vi "Get I2C Channels.vi"(8 "Error In":errorcluster, 11 "LINX Device Config":T1) -> (0 "Error Out":errorcluster, 1 "Num Channels":u8, 2 "I2C Channels":u8[](array[numeric]), 3 "LINX Device Config":T1)   [LabVIEW 2014, in "LMH-LINX.lvlib" / "Device.lvlib"]
uses:
  <vilib>/MakerHub/LINX/Private/Device/Device.lvlib
  <vilib>/MakerHub/LINX/Private/Device/Type Defs/LINX Device Config.ctl
  <vilib>/MakerHub/LINX/Private/Type Defs/Interface.ctl
  <vilib>/MakerHub/LINX/Private/Device/Type Defs/TCP Config.ctl
  <vilib>/MakerHub/LINX/Private/Device/Type Defs/Channels.ctl
  <vilib>/MakerHub/LINX/Private/Type Defs/Error Type.ctl
  <vilib>/MakerHub/LINX/LMH-LINX.lvlib
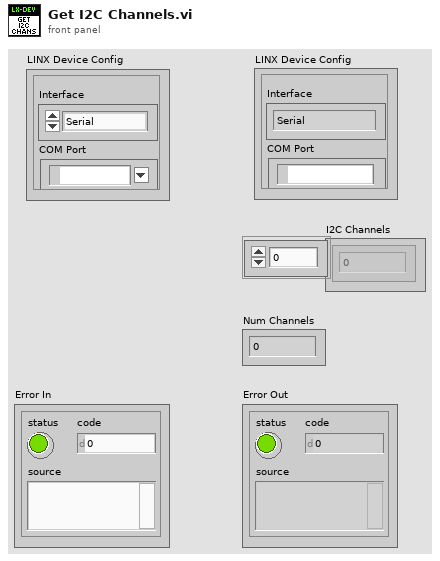
[diagram p1: front panel]
types:
  T1 = typedef "LMH-LINX.lvlib/Device.lvlib/LINX Device Config.ctl" = cluster{"Interface":T2, "COM Port":refnum<visa-resource-name>, "TCP Configuration":T3, "Device Family":u8, "Device ID":u8, "Device Name":string, "TCP Ref":refnum<k5>, "Channels":T4}
  T2 = typedef "LMH-LINX.lvlib/Interface.ctl" = enum16{"Serial", "TCP"}
  T3 = typedef "LMH-LINX.lvlib/Device.lvlib/TCP Config.ctl" = cluster{"IP Address":string, "Port":u16}
  T4 = typedef "LMH-LINX.lvlib/Channels.ctl" = cluster{"DI":u8[], "DO":u8[], "AI":u8[], "AO":u8[], "PWM":u8[], "QE":u8[], "UART":u8[], "I2C 2":u8[], "SPI":u8[], "CAN":u8[], "Servo":u8[], "AI Ref (V)":dbl, "AI Resolution (Bits)":u8, "AO Ref (V)":dbl, "AO Resolution (Bits)":u8}
  T5 = typedef "LMH-LINX.lvlib/Error Type.ctl" = enum16{"Unknown", "Timeout", "Corrupt Return Packet", "Unable To Connect", "Command Not Supported", "Channel DNE", "Invalid COM Config", "Firmware Version Mismatch", "myRIO Support", "CMD Specific Error", "Local IO Not Supported"}
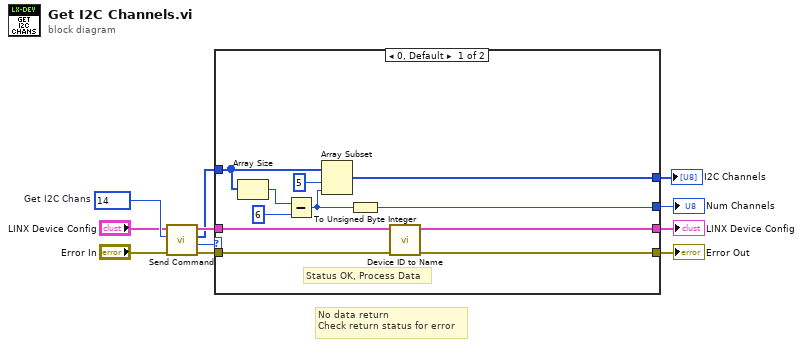
[diagram p0: block diagram]
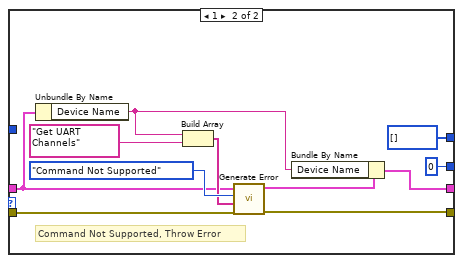
[diagram p2: hidden frame]
diagram:
  w10 = u16 14  # Get I2C Chans
  # "No data return\nCheck return status for error"
  n1 = call <vilib>:"Send Command.vi"("Error In"="Error In", "CMD"=w10, "LINX Device Config"="LINX Device Config") -> ("Error Out"=w5:errorcluster, "Status"=w3:u8, "Response"=w4:u8[], "LINX Device Config"=w7:T1)  [unwired: 5 in]
  n2 = case shown="0, Default" w3 {
    tunnel: [w19 w27] -> w8
    tunnel: w7 -> [w22 w26]
    tunnel: [w20 w32] -> w6
    tunnel: w5 -> [w21 w33]
    tunnel: w4 -> [w18 _]
    tunnel: [w14 u8[] []] -> w2
    tunnel: [w12 u8 0] -> w1
    frame 0, Default {
      # "Status OK, Process Data"
      n3 = Array Size(array=w18) -> (size(s)=w17:i32)
      n4 = Subtract(x=w17, y=6 ("index")) -> (x-y=w13:i32)
      n5 = Array Subset(array=w18, index=5, length=w13) -> (w14:u8[])
      n6 = To Unsigned Byte Integer(number=w13) -> (unsigned 8bit integer=w12:u8)
      n7 = call <vilib>:"Device ID to Name.vi"("Error In"=w21, "LINX Device Config"=w22) -> ("Error Out"=w20:errorcluster, "LINX Device Config"=w19:T1)  [unwired: 7 in, 1 out]
    }
    frame 1 {
      # "Command Not Supported, Throw Error"
      n8 = Unbundle By Name(w26) -> ("Device Name"=w25:string)
      n9 = Build Array(w25, "Get UART Channels") -> (w29:string[])
      n10 = call <vilib>:"Generate Error.vi"("Error In"=w33, "Arguments"=w29, "Error Type"=Error_Type."Command Not Supported", "LINX Device Config"=w26) -> ("Error Out"=w32:errorcluster, "Dup LINX Device Config"=w28:T1)  [unwired: 6 in]
      n11 = Bundle By Name(cluster=w28, "Device Name"=w25) -> (w27:T1)
    }
  }
  "Error Out" <- w6
  "LINX Device Config" <- w8
  "I2C Channels" <- w2
  "Num Channels" <- w1
